vi "MecaKinematics_ToChassisSpeeds.vi"(9 "MECA_WHEEL_SPEEDS":T4 {"RearRightSpeed" format="%19.3f"; "RearLeftSpeed" format="%19.3f"; "FrontRightSpeed" format="%19.3f"; "FrontLeftSpeed" format="%19.3f"}, 11 "in MECA_DRIVE_KINEMATICS":T1={"FrontLeft"={"X"=0.0, "Y"=0.0}, "FrontRight"={"X"=0.0, "Y"=0.0}, "RearLeft"={"X"=0.0, "Y"=0.0}, "RearRight"={"X"=0.0, "Y"=0.0}, "InverseKinematics"=[[0.0, 1.0, -1.0, 0.0], [0.0, 1.0, 1.0, 0.0], [0.0, 1.0, 1.0, 0.0], [0.0, 1.0, -1.0, 0.0]], "ForwardKinematics"=[[0.0, 1.0, -1.0, 0.0], [0.0, 1.0, 1.0, 0.0], [0.0, 1.0, 1.0, 0.0], [0.0, 1.0, -1.0, 0.0]], "PrevCoR"={"X"=0.0, "Y"=0.0}} {"PrevCoR"."Y" format="%14.3f"; "PrevCoR"."X" format="%14.3f"; "RearRight"."Y" format="%14.3f"; "RearRight"."X" format="%14.3f"; "RearLeft"."Y" format="%14.3f"; "RearLeft"."X" format="%14.3f"; "FrontRight"."Y" format="%14.3f"; "FrontRight"."X" format="%14.3f"; "FrontLeft"."Y" format="%14.3f"; "FrontLeft"."X" format="%14.3f"}) -> (1 "ChassisSpeeds":T5 {"vOmega" format="%10.3f"; "vY" format="%10.3f"; "vX" format="%10.3f"})   [LabVIEW 2019, in "Trajectory_Library.lvlib"]
doc: "Performs forward kinematics to return the resulting chassis state from the given wheel speeds. This method is often used for odometry -- determining the robot's position on the field using data from the real-world speed of each wheel on the robot.\n\nParametetrs:\n - MecaDriveKinematics - Data structure\n - WheelSpeeds - The current mecanum drive wheel speeds.\n\nReturns:\n - ChassisSpeeds - The resulting chassis speed."
uses:
  Trajectory_Library.lvlib
  CHASSIS_SPEEDS.ctl
  MECA_WHEEL_SPEEDS.ctl
  MECA_DRIVE_KINEMATICS.ctl
  TRANSLATION2D.ctl
  <vilib>/Analysis/Matrix/Datatypes/RealMatrix.ctl
  <vilib>/Analysis/Matrix/Numeric/Multiply/Multiply - RM,RM.vi
  <vilib>/Analysis/Matrix/NI_Matrix.lvlib
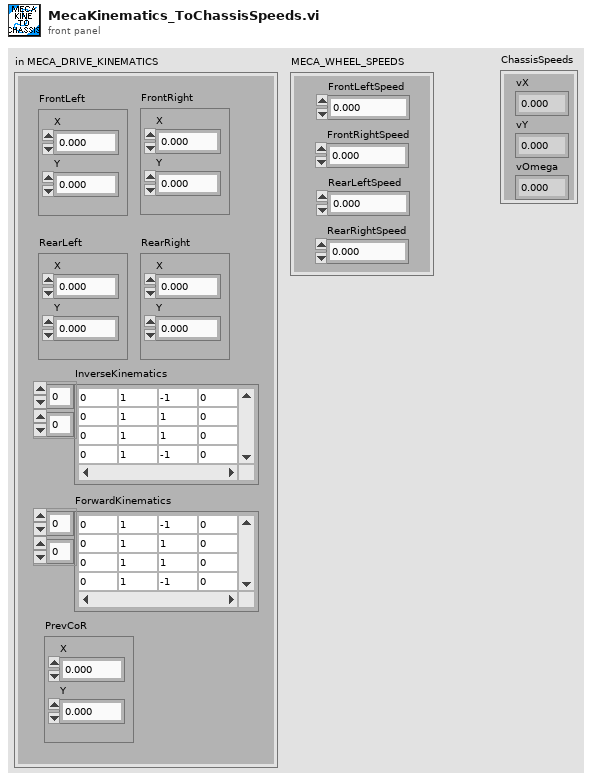
[diagram p1: front panel]
types:
  T1 = typedef "Trajectory_Library.lvlib/MECA_DRIVE_KINEMATICS.ctl" = cluster{"FrontLeft":T2, "FrontRight":T2, "RearLeft":T2, "RearRight":T2, "InverseKinematics":T3, "ForwardKinematics":T3, "PrevCoR":T2}
  T2 = typedef "Trajectory_Library.lvlib/TRANSLATION2D.ctl" = cluster{"X":dbl, "Y":dbl}
  T3 = typedef "NI_Matrix.lvlib/RealMatrix.ctl" = dbl[][]
  T4 = typedef "Trajectory_Library.lvlib/MECA_WHEEL_SPEEDS.ctl" = cluster{"FrontLeftSpeed":dbl, "FrontRightSpeed":dbl, "RearLeftSpeed":dbl, "RearRightSpeed":dbl}
  T5 = typedef "Trajectory_Library.lvlib/CHASSIS_SPEEDS.ctl" = cluster{"vX":dbl, "vY":dbl, "vOmega":dbl}
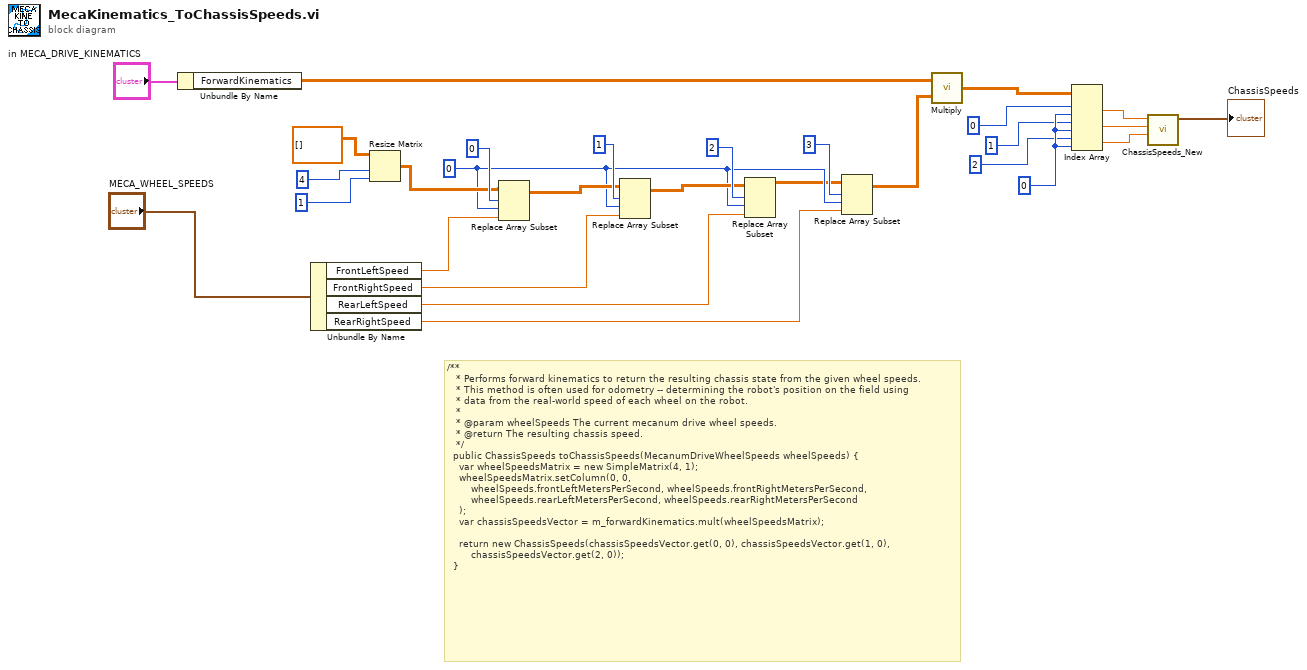
[diagram p0: block diagram]
diagram:
  w20 = 0 ("index (col)")
  w15 = 0 ("disabled index (col)")
  # "/**\n   * Performs forward kinematics to return the resulting chassis state from the given wheel speeds.\n   * This method is often used for odometry -- determining the robot's position on the field using\n   * data from the real-world speed of each wheel on the robot.\n   *\n   * @param wheelSpeeds The current mecanum drive wheel speeds.\n   * @return The resulting chassis speed.\n   */\n  public ChassisSpeeds toChassisSpeeds(MecanumDriveWheelSpeeds wheelSpeeds) {\n    var wheelSpeedsMatrix = new SimpleMatrix(4, 1);\n    wheelSpeedsMatrix.setColumn(0, 0,\n        wheelSpeeds.frontLeftMetersPerSecond, wheelSpeeds.frontRightMetersPerSecond,\n        wheelSpeeds.rearLeftMetersPerSecond, wheelSpeeds.rearRightMetersPerSecond\n    );\n    var chassisSpeedsVector = m_forwardKinematics.mult(wheelSpeedsMatrix);\n\n    return new ChassisSpeeds(chassisSpeedsVector.get(0, 0), chassisSpeedsVector.get(1, 0),\n        chassisSpeedsVector.get(2, 0));\n  }"
  n1 = Unbundle By Name("in MECA_DRIVE_KINEMATICS") -> ("ForwardKinematics"=w7:T3)
  n2 = Unbundle By Name("MECA_WHEEL_SPEEDS") -> ("FrontLeftSpeed"=w12:dbl, "FrontRightSpeed"=w11:dbl, "RearLeftSpeed"=w10:dbl, "RearRightSpeed"=w9:dbl)
  n3 = Resize Matrix(1:1 ("number of columns"), 2:4 ("number of rows"), 4:T3 [] ("matrix")) -> (0:w23:T3)
  n4 = Replace Array Subset(array=w23, new element=w12, index (row)=0 ("disabled index (row)"), index (col)=w15) -> (w22:T3)
  n5 = Replace Array Subset(array=w22, new element=w11, index (row)=1 ("disabled index (row)"), index (col)=w15) -> (w21:T3)
  n6 = Replace Array Subset(array=w21, new element=w10, index (row)=2 ("disabled index (row)"), index (col)=w15) -> (w14:T3)
  n7 = Replace Array Subset(array=w14, new element=w9, index (row)=3 ("disabled index (row)"), index (col)=w15) -> (w6:T3)
  n8 = call-poly <vilib>:"Multiply.vi"("Real Matrix B"=w6, "Real Matrix A"=w7) -> ("A * B"=w5:T3)
  n9 = Index Array(array=w5, index (row) #1=0 ("index (row)"), index (col) #1=w20, index (row) #2=1 ("index (row)"), index (col) #2=w20, index (row) #3=2 ("index (row)"), index (col) #3=w20) -> (element #1=w4:dbl, element #2=w3:dbl, element #3=w2:dbl)
  n10 = call "ChassisSpeeds_New.vi"("vAngular"=w2, "vY"=w3, "vX"=w4) -> ("CHASSIS"=→"ChassisSpeeds":T5)  [unwired: 8 in]
